vi "Example of Loops.vi"() -> ()   [LabVIEW 2016]
uses:
  <vilib>/express/express arith-compare/Formula/XNode/ExpressFormulaBlockNode.xnode
panel:
  out "Formula Block":dbl
  out "Case Statement":string
  out "While Loop 2":dbl
  out "While Loop":dbl
  out "For Loop Output":dbl
  in  "For Loop X":dbl
  # "Examples are from top to bottom in block diagram.\nTo view block diagram, select window->ctr+e or show block diagram."
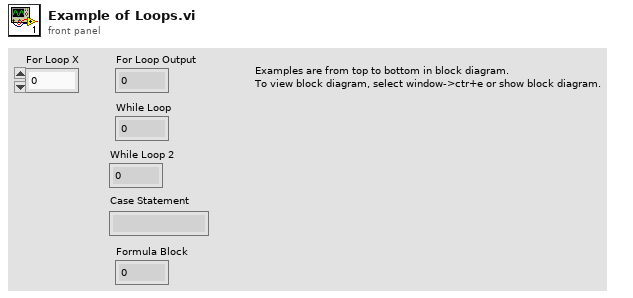
[diagram p1: front panel]
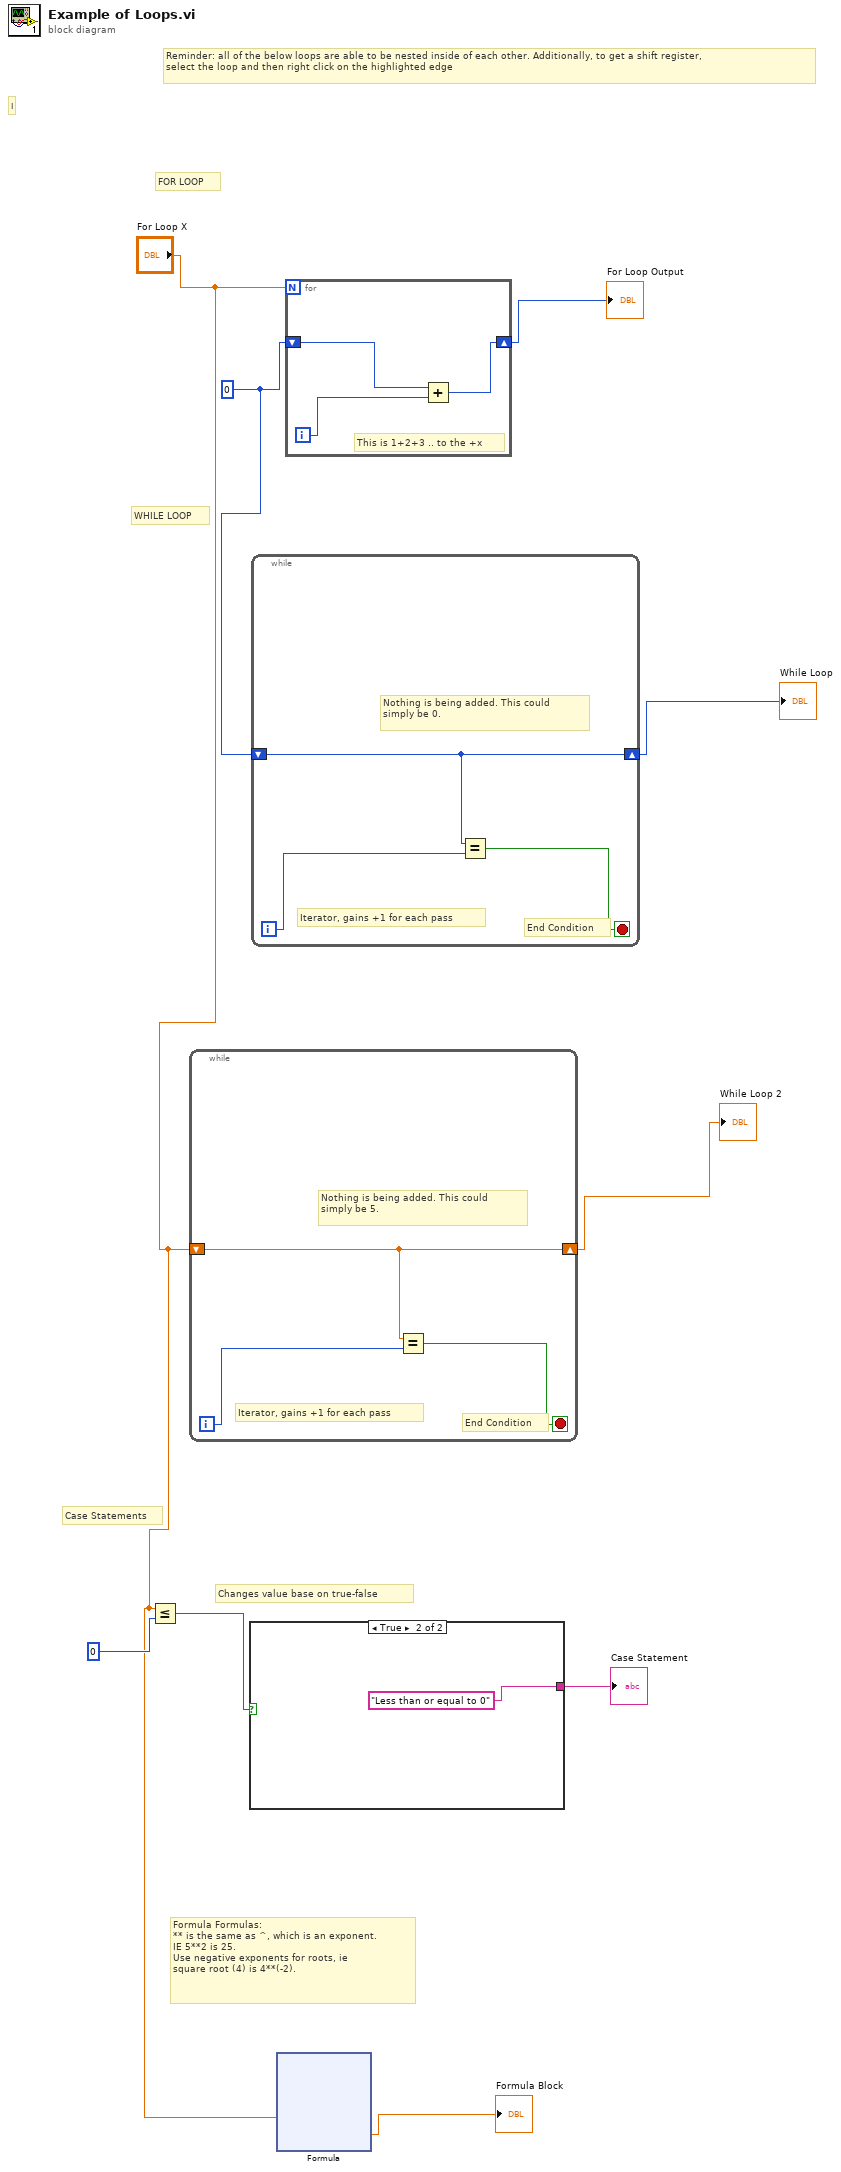
[diagram p0: block diagram]
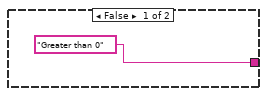
[diagram p2: hidden frame]
diagram:
  w8 = 0
  # "I"
  # "Formula Formulas: \n** is the same as ^, which is an exponent.\nIE 5**2 is 25.\nUse negative exponents for roots, ie\nsquare root (4) is 4**(-2)."
  # "Changes value base on true-false"
  # "Case Statements"
  # "Reminder: all of the below loops are able to be nested inside of each other. Additionally, to get a shift register,\nselect the loop and then right click on the highlighted edge"
  # "WHILE LOOP"
  # "FOR LOOP"
  n1 = Less Or Equal?(x="For Loop X", y=0) -> (x <= y?=w4:bool)
  n2 = while {
    shift-right: [w11] -> w6
    shift-left: "For Loop X" -> [w11]
    i -> [w12]
    stop <- w10 stop-if-true
    # "Nothing is being added. This could\nsimply be 5."
    # "Iterator, gains +1 for each pass"
    # "End Condition"
    n3 = Equal?(x=w11, y=w12) -> (x = y?=w10:bool)
  }
  "While Loop 2" <- w6
  n4 = case shown="True" w4 {
    tunnel: ["Greater than 0" "Less than or equal to 0"] -> w3
    frame False {
    }
    frame True {
    }
  }
  "Case Statement" <- w3
  n5 = while {
    shift-right: [w16] -> w7
    shift-left: w8 -> [w16]
    i -> [w17]
    stop <- w15 stop-if-true
    # "Nothing is being added. This could\nsimply be 0."
    # "Iterator, gains +1 for each pass"
    # "End Condition"
    n6 = Equal?(x=w16, y=w17) -> (x = y?=w15:bool)
  }
  "While Loop" <- w7
  n7 = xnode "Formula"("X1"="For Loop X") -> ("Result"=→"Formula Block":dbl)  [unwired: 1 in, 1 out]
  n8 = for {
    N: "For Loop X" -> [_]
    shift-right: [w18] -> w9
    shift-left: w8 -> [w19]
    i -> [w20]
    # "This is 1+2+3 .. to the +x"
    n9 = Add(x=w19, y=w20) -> (x+y=w18:i32)
  }
  "For Loop Output" <- w9
